vi "Write NS (HMI).vi"(8 "error in (no error)":errorcluster, 10 "Message Data":variant, 11 "Message":string) -> (0 "error out":errorcluster)   [LabVIEW 2021]
uses:
  support/Message Queue/Message Cluster.ctl
  GV/HMI GV.vi
  support/Message Queue/Message Queue.lvlib
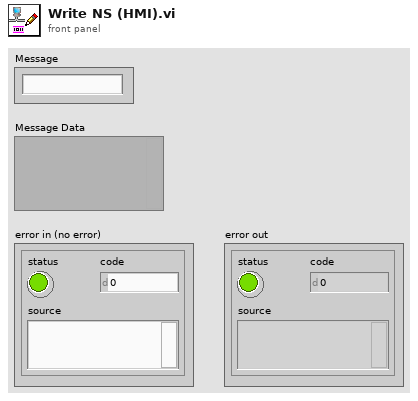
[diagram p1: front panel]
types:
  T1 = typedef "Message Queue.lvlib/Message Cluster.ctl" = cluster{"Message":string, "Message Data":variant}
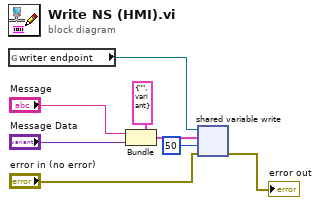
[diagram p0: block diagram]
diagram:
  n1 = global read "HMI GV.vi" "writer endpoint"() -> (w1:refnum<k21>)
  n2 = Bundle(cluster=T1 {"Message"="", "Message Data"=variant} ("Message Cluster"), "Message"="Message", "Message Data"="Message Data") -> (w4:T1)
  n3 = shared-variable-write(w1, "error in (no error)", w4, 50 ("timeout ms (-1)")) -> (→"error out":errorcluster)  [unwired: 2 out]
